vi "daily_total.vi"(0 "Input array":dbl[][](array[numeric])) -> (1 "Daily totals (MJ d-1 m-2)":dbl[](array[numeric]), 2 "Yearly total (GJ d-1 m-2)":dbl)   [LabVIEW 2012]
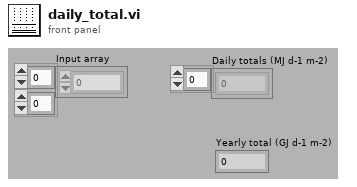
[diagram p1: front panel]
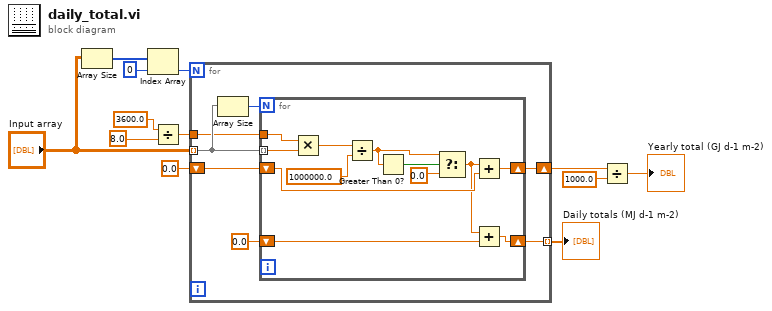
[diagram p0: block diagram]
diagram:
  n1 = Array Size(array="Input array") -> (size(s)=w12:i32[])
  n2 = Index Array(array=w12, index=0) -> (element=w11:i32)
  n3 = Divide(x=3600.0, y=8.0) -> (x/y=w4:dbl)
  n4 = for {
    N: w11 -> [_]
    tunnel: "Input array" -> [w18] mode=indexing
    tunnel: [w16] -> w8 mode=indexing
    shift-right: [w14] -> w3
    shift-left: 0.0 -> [w15]
    tunnel: w4 -> [w13]
    n5 = Array Size(array=w18) -> (size(s)=w19:i32)
    n6 = for {
      N: w19 -> [_]
      tunnel: w18 -> [w25] mode=indexing
      shift-right: [w30] -> w16
      shift-left: 0.0 -> [w31]
      shift-right: [w28] -> w14
      shift-left: w15 -> [w29]
      tunnel: w13 -> [w24]
      n7 = Multiply(x=w24, y=w25) -> (x*y=w27:dbl)
      n8 = Divide(x=w27, y=1000000.0) -> (x/y=w22:dbl)
      n9 = Greater Than 0?(x=w22) -> (x > 0?=w23:bool)
      n10 = Select(t=w22, s=w23, f=0.0) -> (s? t:f=w21:dbl)
      n11 = Add(x=w21, y=w29) -> (x+y=w28:dbl)
      n12 = Add(x=w21, y=w31) -> (x+y=w30:dbl)
    }
  }
  "Daily totals (MJ d-1 m-2)" <- w8
  n13 = Divide(x=w3, y=1000.0) -> (x/y=→"Yearly total (GJ d-1 m-2)":dbl)
